vi "c_ctre_phoenix6_encode_device.vi"(0 "Numeric 2":i32, 1 "String 2":string, 2 "String 4":string, 3 "Numeric 4":u32) -> (20 "Numeric":i32, 21 "String":string, 22 "String 3":string, 23 "Numeric 3":u32)   [LabVIEW 2023]
uses:
  <vilib>/Rock Robotics/WPI/ThirdParty/Phoenix-LabVIEW/Controls/DriverLib.ctl
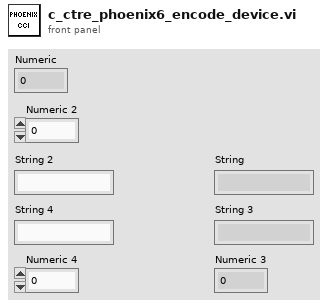
[diagram p1: front panel]
types:
  T1 = typedef "DriverLib.ctl" = path
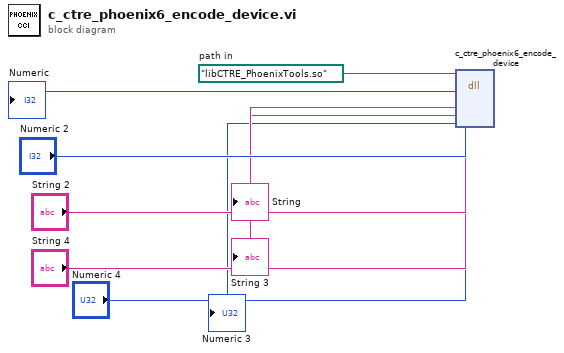
[diagram p0: block diagram]
diagram:
  w9 = T1 path "libCTRE_PhoenixTools.so"  # path in
  n1 = dll-call lib="?" fn="c_ctre_phoenix6_encode_device"(path in=w9, "Numeric 2", "String 2", "String 4", "Numeric 4") -> (→"Numeric":i32, →"String":string, →"String 3":string, →"Numeric 3":u32)  [unwired: 3 in, 2 out]
